vi "WPI_PWMSafetyConfig.vi"(8 "error in (no error)":errorcluster, 9 "timeout (s)":dbl=0.1, 10 "mode":T1, 11 "PWMDeviceRef":T2={"DeviceStatus"={"status"=FALSE, "code"=0, "source"=""}, "PWM Channel"=enum."PWM 1"}) -> (0 "error out":errorcluster, 3 "PWMDeviceRef":T2={"DeviceStatus"={"status"=FALSE, "code"=0, "source"=""}, "PWM Channel"=enum."PWM 1"})   [LabVIEW 2017]
doc: "Turns off PWM if PWM does not receive updates faster than the <b>timeout (s)</b> value. This VI is a safety feature to ensure the robot responds to input values, such as joystick values.\n\nThis software is licensed. Open the labview\\readme\\WPI Robotics Library Open Source License.txt file for more information."
uses:
  <vilib>/Rock Robotics/WPI/PWM/WPI_PWMDeviceRef.ctl
  <vilib>/Rock Robotics/SystemInterfaces/DIO/FPGA_DIOPWMChannel.ctl
  <vilib>/Rock Robotics/WPI/SafetyOutput/WPI_SafetyOutputConfigMenu.ctl
  <vilib>/Rock Robotics/WPI/SafetyOutput/WPI_SafetyOutputCheckMenu.ctl
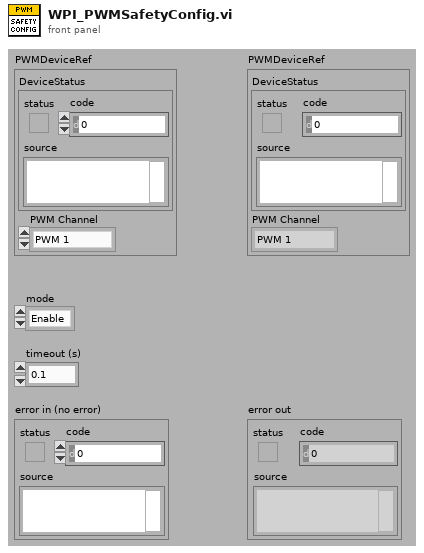
[diagram p1: front panel]
types:
  T1 = typedef "WPI_SafetyOutputConfigMenu.ctl" = enum16{"Enable", "Disable"}
  T2 = typedef "WPI_PWMDeviceRef.ctl" = cluster{"DeviceStatus":errorcluster, "PWM Channel":T3}
  T3 = typedef "FPGA_DIOPWMChannel.ctl" = enum8{"PWM 0", "PWM 1", "PWM 2", "PWM 3", "PWM 4", "PWM 5", "PWM 6", "PWM 7", "PWM 8", "PWM 9", "PWM MXP 0", "PWM MXP 1", "PWM MXP 2", "PWM MXP 3", "PWM MXP 4", "PWM MXP 5", "PWM MXP 6", "PWM MXP 7", "PWM MXP 8", "PWM MXP 9", "Invalid"}
  T4 = typedef "WPI_SafetyOutputCheckMenu.ctl" = enum16{"test", "add", "remove", "update"}
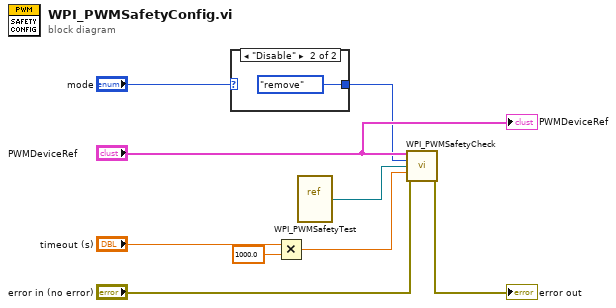
[diagram p0: block diagram]
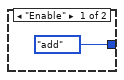
[diagram p2: hidden frame]
diagram:
  n1 = case shown="\"Disable\"" "mode" {
    tunnel: [WPI_SafetyOutputCheckMenu."add" ("menu") WPI_SafetyOutputCheckMenu."remove" ("menu")] -> w4
    frame "Enable" {
    }
    frame "Disable" {
    }
  }
  n2 = Multiply(x="timeout (s)", y=1000.0) -> (x*y=w2:dbl)
  n3 = vi-ref <vilib>:"WPI_PWMSafetyTest.vi"() -> (w3:refnum<vi>)
  n4 = call <vilib>:"WPI_PWMSafetyCheck.vi"("PWMDeviceRef"="PWMDeviceRef", "menu"=w4, "VI Refnum"=w3, "timeout (ms)"=w2, "error in (no error)"="error in (no error)") -> ("error out"=→"error out":errorcluster)  [unwired: 10 out]
  "PWMDeviceRef" <- "PWMDeviceRef"
